vi "Write Energy.vi"(8 "error in (no error)":errorcluster, 10 "Energy":dbl[unit]=10.0, 11 "POLARIS Target Focus Actor in":refnum<class "POLARIS Target Focus Actor.lvclass">) -> (0 "error out":errorcluster, 3 "POLARIS Target Focus Actor out":refnum<class "POLARIS Target Focus Actor.lvclass">)   [LabVIEW 2014, in "POLARIS Target Focus Actor.lvlib" / "POLARIS Target Focus Actor.lvclass"]
uses:
  POLARIS Target Focus Actor.lvclass
  POLARIS Target Focus Actor.lvclass/POLARIS Target Focus Actor.ctl
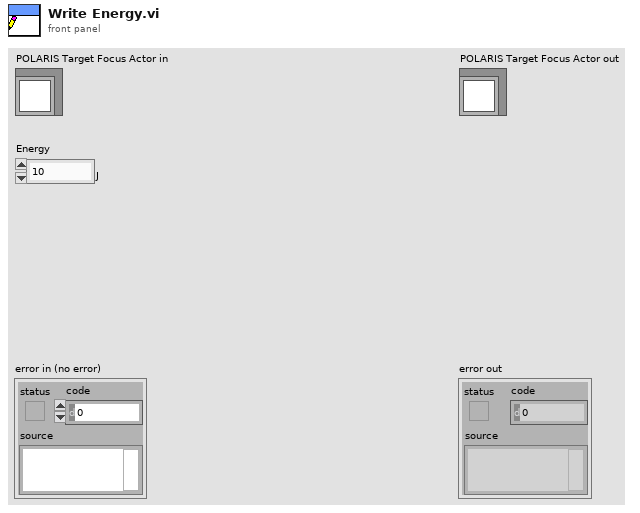
[diagram p1: front panel]
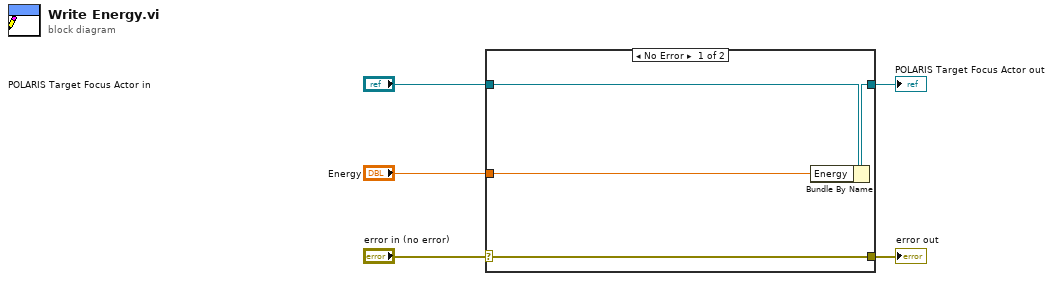
[diagram p0: block diagram]
diagram:
  n1 = case shown="No Error" "error in (no error)" {
    selector: "error in (no error)" -> [w9 w10]
    tunnel: [w9 w10] -> w4
    tunnel: [w7 w11] -> w2
    tunnel: "POLARIS Target Focus Actor in" -> [w8 w11]
    tunnel: "Energy" -> [w6 _]
    frame No Error {
      n2 = Bundle By Name(cluster=w8, "Energy"=w6) -> (w7:refnum<class "POLARIS Target Focus Actor.lvclass">)
    }
    frame Error {
    }
  }
  "error out" <- w4
  "POLARIS Target Focus Actor out" <- w2
